vi "Pressure auto-adjust background loop.vi"(10 "Target pressure range":T1, 11 "Pressure Control in":refnum<class "Pressure Control.lvclass">) -> ()   [LabVIEW 2014, in "Pressure Control.lvclass"]
uses:
  Pressure Control.lvclass
  Auto-adjust Pressure Range.ctl
panel:
  in  "Stop":bool
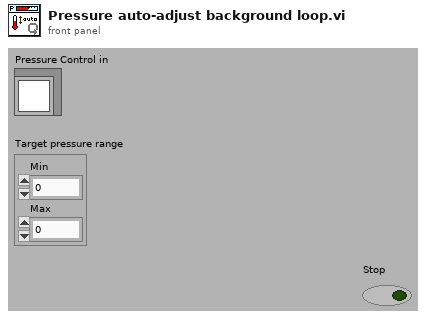
[diagram p1: front panel]
types:
  T1 = typedef "Pressure Control.lvclass/Auto-adjust Pressure Range.ctl" = cluster{"Min":dbl, "Max":dbl}
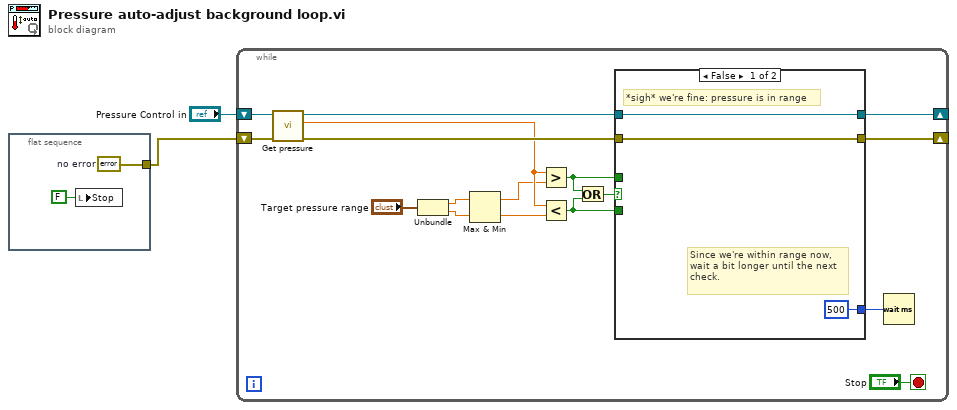
[diagram p0: block diagram]
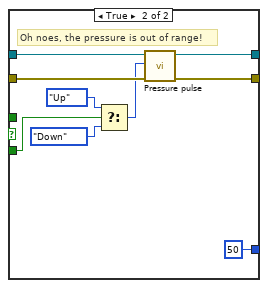
[diagram p2: hidden frame]
diagram:
  n1 = flat-sequence {
    tunnel: [w3] -> w1
    frame #0 {
      w3 = errorcluster {"status"=FALSE, "code"=0, "source"=""}  # no error
      n2 = local write "Stop"(FALSE ("Stop")) -> ()
    }
  }
  n3 = while {
    shift-right: [w16] -> _
    shift-left: "Pressure Control in" -> [w20]
    shift-right: [w11] -> _
    shift-left: w1 -> [w10]
    stop <- "Stop" stop-if-true
    n4 = call "Get pressure.vi"("error in (no error)"=w10, "Pressure Control in"=w20) -> ("error out"=w21:errorcluster, "Pressure"=w18:dbl, "Pressure Control out"=w15:refnum<class "Pressure Control.lvclass">)  [unwired: 6 in, 1 out]
    n5 = Unbundle("Target pressure range") -> ("Min"=w9:dbl, "Max"=w8:dbl)
    n6 = Max & Min(x=w9, y=w8) -> (max(x,y)=w6:dbl, min(x,y)=w7:dbl)
    n7 = Greater?(x=w18, y=w6) -> (0:w12:bool)
    n8 = Less?(x=w18, y=w7) -> (x < y?=w13:bool)
    n9 = Or(x=w12, y=w13) -> (x .or. y?=w17:bool)
    n10 = case shown="False" w17 {
      tunnel: [w24 w29] -> w16
      tunnel: w15 -> [w24 w30]
      tunnel: [u32 500 u32 50] -> w14
      tunnel: w13 -> [_ w31]
      tunnel: w12 -> [_ _]
      tunnel: w21 -> [w22 w33]
      tunnel: [w22 w25] -> w11
      frame False {
        # "Since we're within range now, wait a bit longer until the next check."
        # "*sigh* we're fine: pressure is in range"
      }
      frame True {
        # "Oh noes, the pressure is out of range!"
        n11 = Select(t=enum16{"Up", "Down"}."Up" ("Up or down?"), s=w31, f=enum16{"Up", "Down"}."Down" ("Up or down?")) -> (s? t:f=w26:enum16{"Up", "Down"})
        n12 = call "Pressure pulse.vi"("error in (no error)"=w33, "Up or down?"=w26, "Pressure Control in"=w30) -> ("error out"=w25:errorcluster, "Pressure Control out"=w29:refnum<class "Pressure Control.lvclass">)  [unwired: 7 in]
      }
    }
    n13 = Wait (ms)(milliseconds to wait=w14) -> ()  [unwired: 1 out]
  }
